vi "Add Panel Tier.vi"(8 "Error In":errorcluster, 9 "Old VI's Destination":refnum<class "Panel.lvclass"> caption="Replaced Tier's Panel (no panel)", 10 "New VI Ref":refnum<vi> caption="New VI Ref (caller)", 11 "Panel Actor in":refnum<class "Panel Actor.lvclass">) -> (0 "Error Out":errorcluster, 3 "Panel Actor out":refnum<class "Panel Actor.lvclass">)   [LabVIEW 2023, in "Panel Actor.lvlib" / "Panel Actor.lvclass"]
doc: "Adds a new Tier to the panel. Use Panel Tiers to dynamically build UIs that reflect the inheritance of the actor.\n\nWire a VI into <b>New VI Ref</b> to replace VI with a different one.\n\nWire <b>Replaced Tier's Panel</b> to insert the replaced VI in another panel.\n\nThis is useful when creating dynamic UIs that have layers at each chain in the override list. Each parent can use this VI to insert themselves at the base tier, and insert the last layer in a subpanel, for example.\n\nSee the \"Tiered Panel\" example for more information.\n\n<B>Panel Actor In:</B> Panel Actor object.\n<B>New VI Ref:</B> VI reference for the new vi.\n<B>Replaced Tier's Panel:</B> Panel object for the replaced tier.\n<B>Error In:</B> Describes error conditions that occur before this node runs.\n\n<B>Panel Actor Out:</B> Panel Actor object.\n<B>Error Out:</B> Contains error information.\n----\nPlease see the following web address for additional documentation and tutorial information:\nhttp://www.mooregoodideas.com/mgi-panel-manager/\n\nAuthor: Derek Trepanier\n\nCopyright (c) 2018, Moore Good Ideas, Inc.\n\nAll rights reserved.\n\nRedistribution and use in source and binary forms, with or without modification, are permitted provided that the following conditions are met:\n\n * Redistributions of source code must retain the above copyright notice, this list of conditions and the following disclaimer.\n * Redistributions in binary form must reproduce the above copyright notice, this list of conditions and the following disclaimer in the documentation and/or other materials provided with the distribution.\n * Neither the name of Moore Good Ideas, Inc. nor the names of its contributors may be used to endorse or promote products derived from this software without specific prior written permission.\n\nTHIS SOFTWARE IS PROVIDED BY THE COPYRIGHT HOLDERS AND CONTRIBUTORS \"AS IS\" AND ANY EXPRESS OR IMPLIED WARRANTIES, INCLUDING, BUT NOT LIMITED TO, THE IMPLIED WARRANTIES OF MERCHANTABILITY AND FITNESS FOR A PARTICULAR PURPOSE ARE DISCLAIMED. IN NO EVENT SHALL THE COPYRIGHT OWNER OR CONTRIBUTORS BE LIABLE FOR ANY DIRECT, INDIRECT, INCIDENTAL, SPECIAL, EXEMPLARY, OR CONSEQUENTIAL DAMAGES (INCLUDING, BUT NOT LIMITED TO, PROCUREMENT OF SUBSTITUTE GOODS OR SERVICES; LOSS OF USE, DATA, OR PROFITS; OR BUSINESS INTERRUPTION) HOWEVER CAUSED AND ON ANY THEORY OF LIABILITY, WHETHER IN CONTRACT, STRICT LIABILITY, OR TORT (INCLUDING NEGLIGENCE OR OTHERWISE) ARISING IN ANY WAY OUT OF THE USE OF THIS SOFTWARE, EVEN IF ADVISED OF THE POSSIBILITY OF SUCH DAMAGE."
uses:
  Library/Panel Actor.lvclass
  Panel/Panel/Panel.lvclass
  Library/Panel Actor.lvclass/Panel Actor.ctl
  <vilib>/Utility/error.llb/Error Cluster From Error Code.vi
  <vilib>/ErrorRing/Error Ring.xnode
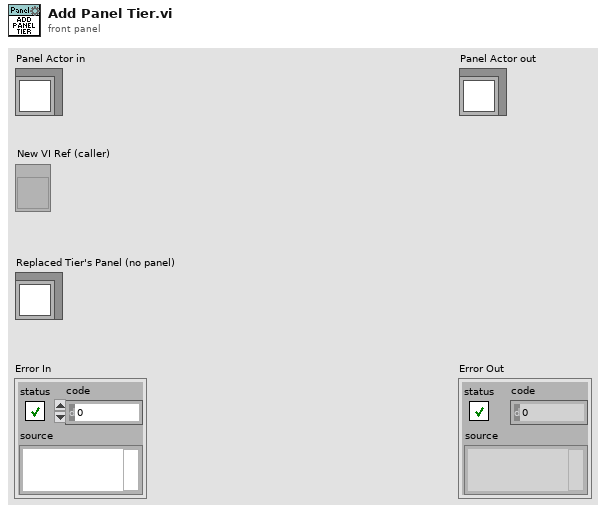
[diagram p1: front panel]
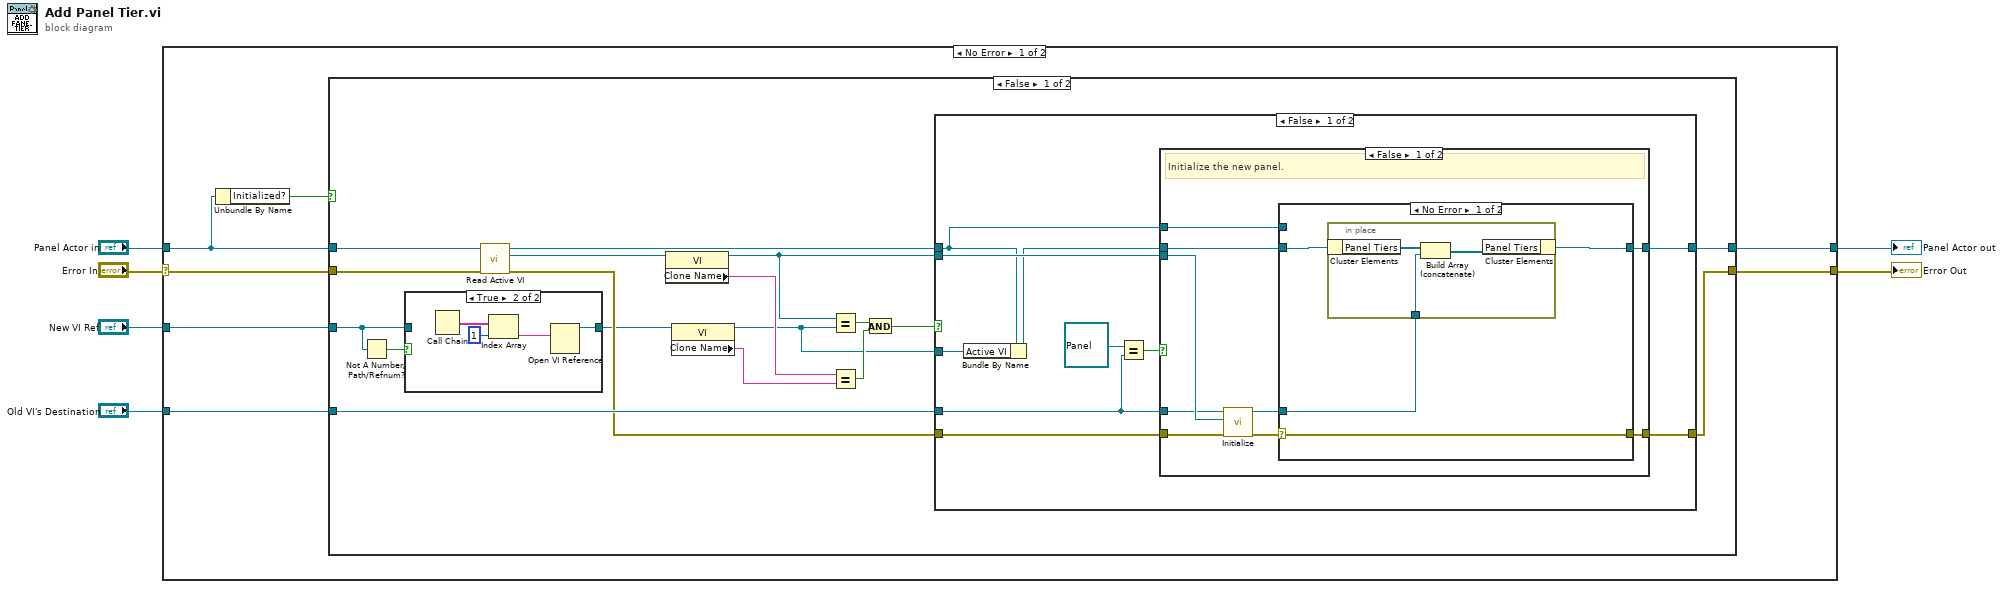
[diagram p0: block diagram]
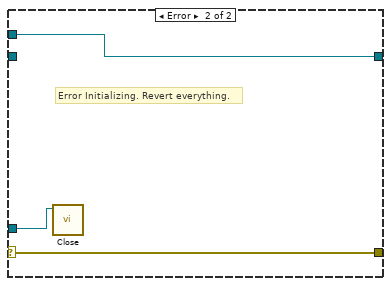
[diagram p3: hidden frame]
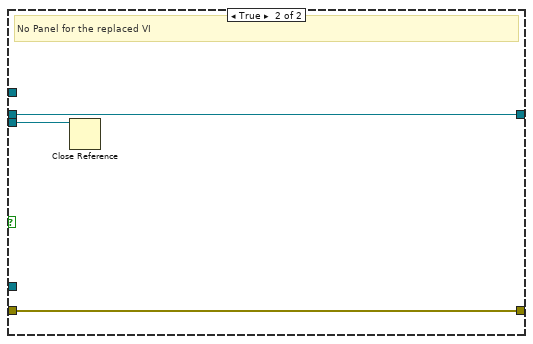
[diagram p4: hidden frame]
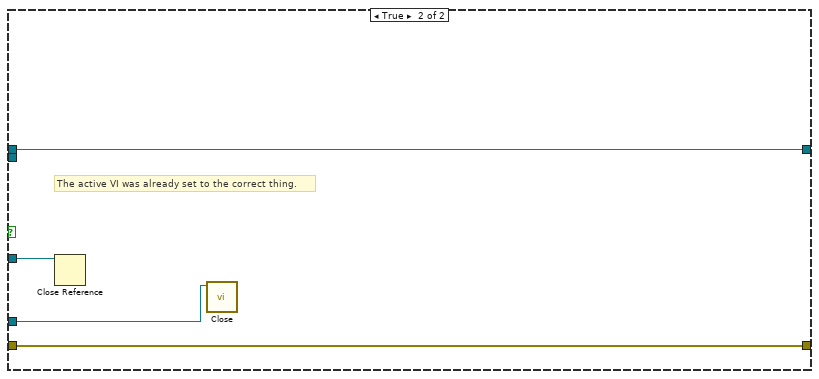
[diagram p5: hidden frame]
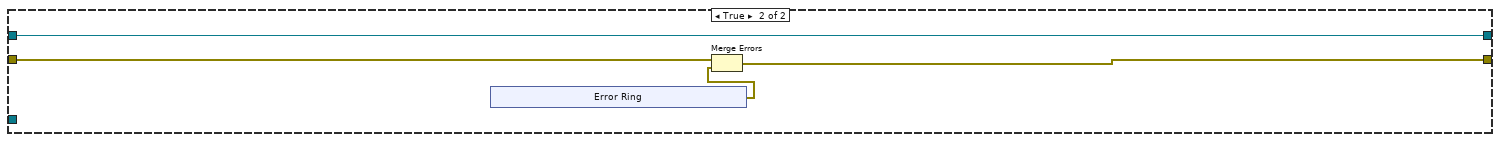
[diagram p6: hidden frame]
diagram:
  n1 = case shown="No Error" "Error In" {
    selector: "Error In" -> [w13 w83]
    tunnel: [w10 w83] -> w5
    tunnel: [w9 w82] -> w3
    tunnel: "Panel Actor in" -> [w8 w82]
    tunnel: "New VI Ref" -> [w11 _]
    tunnel: "Old VI's Destination" -> [w12 _]
    frame No Error {
      n2 = Unbundle By Name(w8) -> ("Initialized?"=w7:bool)
      n3 = case shown="False" w7 {
        tunnel: w13 -> [w30 w75]
        tunnel: w12 -> [w29 _]
        tunnel: w11 -> [w26 _]
        tunnel: [w16 w74] -> w10
        tunnel: w8 -> [w15 w76]
        tunnel: [w14 w76] -> w9
        frame False {
          n4 = Not A Number/Path/Refnum?(number/path/refnum=w26) -> (NaN/Path/Refnum?=w27:bool)
          n5 = case shown="True" w27 {
            tunnel: w26 -> [w32 _]
            tunnel: [w32 w33] -> w22
            frame False {
            }
            frame True {
              n6 = Call Chain() -> (call chain=w36:string[])
              n7 = Index Array(array=w36, index=1) -> (element=w34:string)
              n8 = Open VI Reference(vi path=w34) -> (vi reference=w33:refnum<vi>)  [unwired: 5 in, 1 out]
            }
          }
          n9 = call "Read Active VI.vi"("error in (no error)"=w30, "Panel Actor in"=w15) -> ("error out"=w28:errorcluster, "Active VI ref"=w23:refnum<vi>, "Panel Actor out"=w31:refnum<class "Panel Actor.lvclass">)  [unwired: 7 in]
          n10 = property class="VI"(reference=w23) -> (reference out=w17:refnum<vi>, "Clone Name"=w21:string)  [unwired: 1 in, 1 out]
          n11 = property class="VI"(reference=w22) -> (reference out=w18:refnum<vi>, "Clone Name"=w20:string)  [unwired: 1 in, 1 out]
          n12 = Equal?(x=w17, y=w18) -> (x = y?=w25:bool)
          n13 = Equal?(x=w21, y=w20) -> (x = y?=w19:bool)
          n14 = And(x=w25, y=w19) -> (x .and. y?=w24:bool)
          n15 = case shown="False" w24 {
            tunnel: w29 -> [w40 w69]
            tunnel: w28 -> [w46 w71]
            tunnel: [w45 w71] -> w16
            tunnel: w31 -> [w37 w72]
            tunnel: [w44 w72] -> w14
            tunnel: w18 -> [w41 w70]
            tunnel: w17 -> [w43 _]
            frame False {
              n16 = Bundle By Name(cluster=w37, "Active VI"=w41) -> (w42:refnum<class "Panel Actor.lvclass">)
              n17 = Equal?(x=refnum<class "Panel.lvclass"> refnum, y=w40) -> (x = y?=w38:bool)
              n18 = case shown="False" w38 {
                tunnel: w46 -> [w55 w67]
                tunnel: [w48 w67] -> w45
                tunnel: [w54 w68] -> w44
                tunnel: w43 -> [w53 w66]
                tunnel: w42 -> [w52 w68]
                tunnel: w40 -> [w51 _]
                tunnel: w37 -> [w47 _]
                frame False {
                  # "Initialize the new panel."
                  n19 = call "Initialize.vi"("error in (no error)"=w55, "VI Refnum"=w53, "Panel In"=w51) -> ("error out"=w49:errorcluster, "Panel Out"=w50:refnum<class "Panel.lvclass">)  [unwired: 6 in, 1 out]
                  n20 = case shown="No Error" w49 {
                    selector: w49 -> [w56 w63]
                    tunnel: [w59 w65] -> w54
                    tunnel: w52 -> [w58 _]
                    tunnel: w50 -> [w57 w64]
                    tunnel: [w56 w63] -> w48
                    tunnel: w47 -> [_ w65]
                    frame No Error {
                      n21 = in-place {
                        in-place-border: w57 -> [w60]
                        n22 = in-place-cluster #1(w58) -> ("Panel Tiers"=w62:refnum<class "Panel.lvclass">[])
                        n23 = Build Array (concatenate)(w62, w60) -> (w61:refnum<class "Panel.lvclass">[])
                        n24 = in-place-cluster #1("Panel Tiers"=w61) -> (w59:refnum<class "Panel Actor.lvclass">)
                      }
                    }
                    frame Error {
                      # "Error Initializing. Revert everything."
                      n25 = call-dynamic "Close.vi"("Panel In"=w64) -> ()  [unwired: 10 in, 1 out]
                    }
                  }
                }
                frame True {
                  # "No Panel for the replaced VI"
                  n26 = Close Reference(reference=w66) -> ()  [unwired: 1 in, 1 out]
                }
              }
            }
            frame True {
              # "The active VI was already set to the correct thing."
              n27 = Close Reference(reference=w70) -> ()  [unwired: 1 in, 1 out]
              n28 = call-dynamic "Close.vi"("Panel In"=w69) -> ()  [unwired: 10 in, 1 out]
            }
          }
        }
        frame True {
          n29 = xnode "Error Ring"() -> ("error out"=w73:errorcluster)
          n30 = Merge Errors(w75, w73) -> (w74:errorcluster)
        }
      }
    }
    frame Error {
    }
  }
  "Error Out" <- w5
  "Panel Actor out" <- w3
